vi "crop_roi.vi"(1 "Refnum in":T1, 2 "Roy Radius":dbl, 3 "Y":dbl, 4 "X":dbl) -> (0 "Refnum in 2":T1)   [LabVIEW 2014]
uses:
  <vilib>/vision/Image Controls.llb/IMAQ Image.ctl
  <vilib>/vision/NI_Vision_Development_Module.lvlib
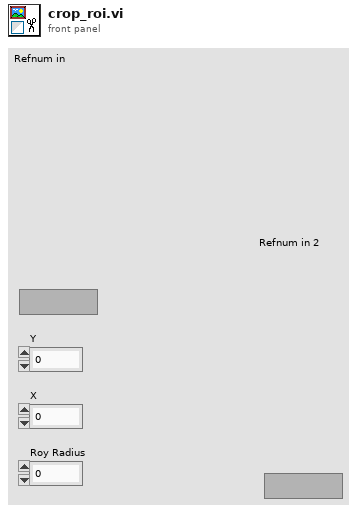
[diagram p1: front panel]
types:
  T1 = typedef "IMAQ Image.ctl" = refnum<image>
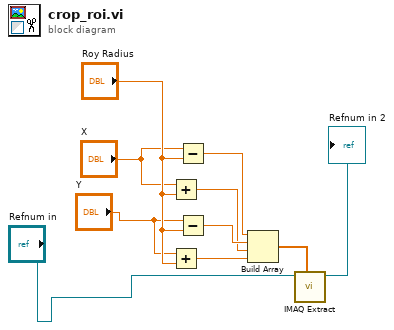
[diagram p0: block diagram]
diagram:
  n1 = Add(x="X", y="Roy Radius") -> (x+y=w2:dbl)
  n2 = Add(x="Y", y="Roy Radius") -> (x+y=w5:dbl)
  n3 = Subtract(x="X", y="Roy Radius") -> (x-y=w4:dbl)
  n4 = Subtract(x="Y", y="Roy Radius") -> (x-y=w6:dbl)
  n5 = Build Array(w4, w6, w2, w5) -> (w3:dbl[])
  n6 = call "IMAQ Extract"("Optional Rectangle"=w3, "Image Src"="Refnum in") -> ("Image Dst Out"=→"Refnum in 2":T1)  [unwired: 8 in, 1 out]
